vi "getObservers.vi"(8 "error in (no error)":errorcluster, 11 "WeatherData in":refnum<class "WeatherData.lvclass">) -> (0 "error out":errorcluster, 2 "Observers":refnum<class "Observer.lvclass">[](array[class]), 3 "WeatherData out":refnum<class "WeatherData.lvclass">)   [LabVIEW 2017, in "WeatherData.lvclass"]
uses:
  WeatherData.lvclass
  Observer/Observer.lvclass
  Observable/Observable.lvclass
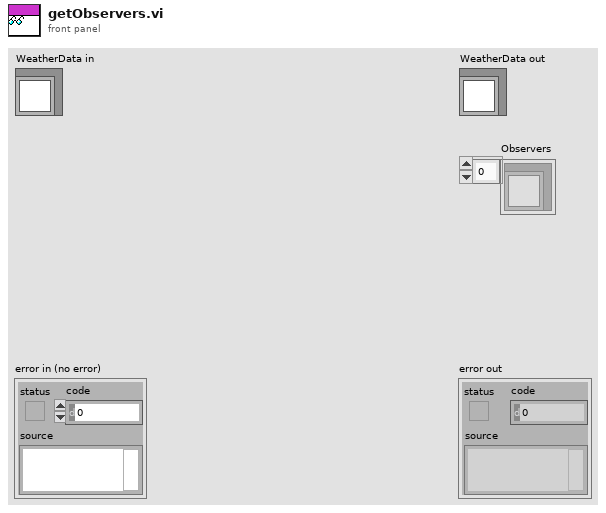
[diagram p1: front panel]
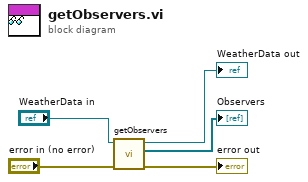
[diagram p0: block diagram]
diagram:
  n1 = call-parent "getObservers.vi"("error in (no error)"="error in (no error)", "Observable in"="WeatherData in") -> ("error out"=→"error out":errorcluster, "Observers"=→"Observers":refnum<class "Observer.lvclass">[], "Observable out"=→"WeatherData out":refnum<class "WeatherData.lvclass">)  [unwired: 7 in]
